vi "Test JSON config.vi"(0 "request cluster":variant, 1 "command description":string, 2 "command":string, 5 "<JSON> request documentation":string, 7 "response cluster":variant, 9 "<JSON> response documentation":string, 11 "error in (no error)":errorcluster) -> (4 "<JSON> API documentation":string, 15 "error out":errorcluster)   [LabVIEW 2019, in "Instrument.lvlib" / "Instrument.lvclass"]
uses:
  Instrument.lvclass
  ca868cea-1423-40d0-bede-52914c02769a.vi
  47e4b0b2-8925-4823-9c6b-443795284c27.vi
  <vilib>/JDP Science/JSONtext/Variant to JSON Text.vi
  <vilib>/JDP Science/JSONtext/LVClass Serializer/JSONtext LVClass Serializer.lvclass
  <vilib>/JDP Science/JSONtext/JSONtext.lvlib
  subsystems/Help/Help.lvclass
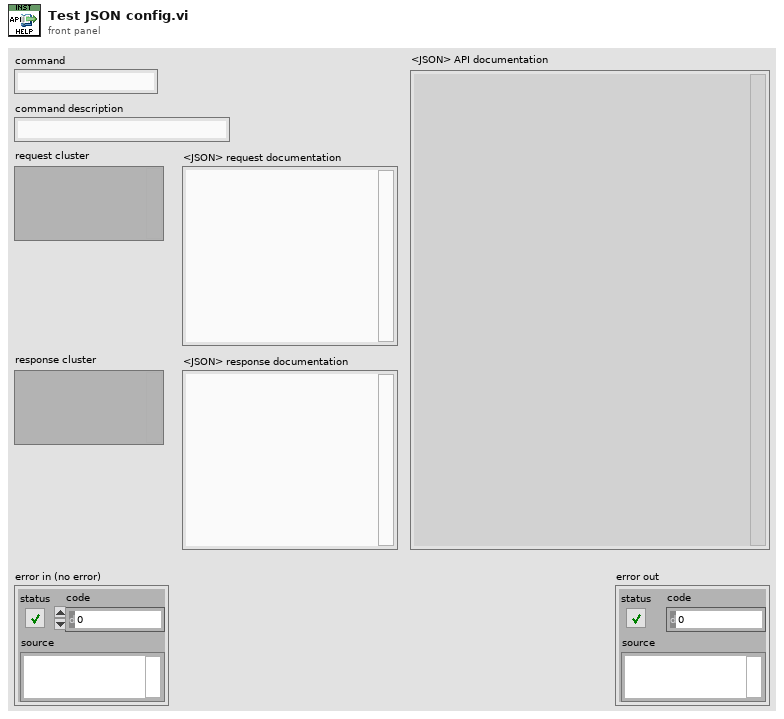
[diagram p1: front panel]
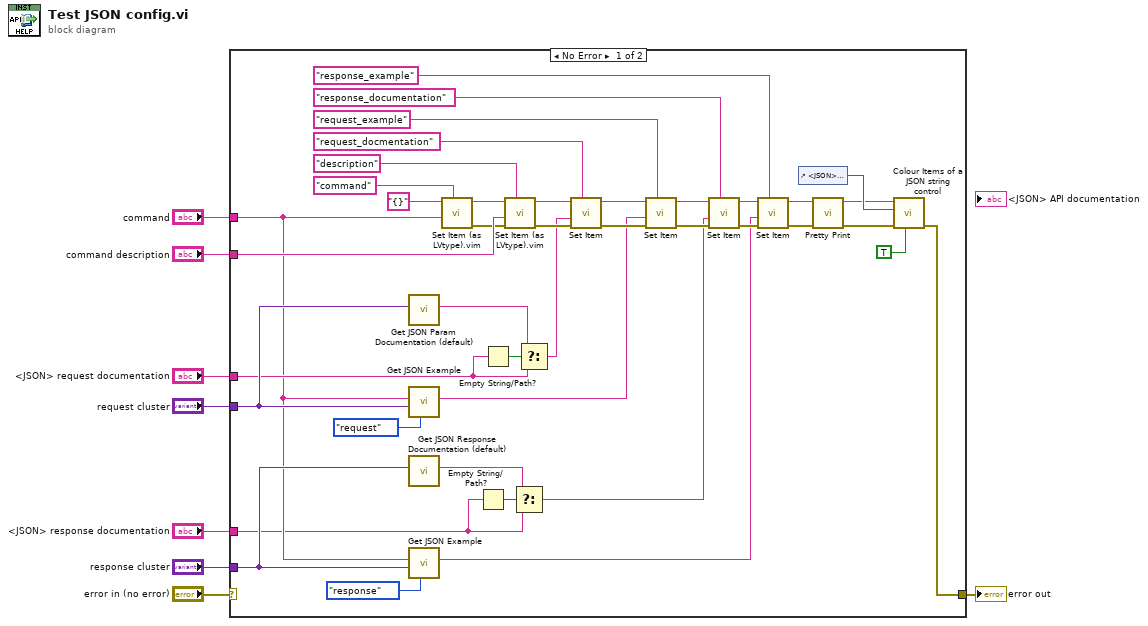
[diagram p0: block diagram]
diagram:
  n1 = case shown="No Error" "error in (no error)" {
    selector: "error in (no error)" -> [_ w49]
    tunnel: "command" -> [w14 _]
    tunnel: "command description" -> [w27 _]
    tunnel: "request cluster" -> [w41 _]
    tunnel: "<JSON> request documentation" -> [w38 _]
    tunnel: [w28 w49] -> w4
    tunnel: "response cluster" -> [w15 _]
    tunnel: "<JSON> response documentation" -> [w9 _]
    frame No Error {
      n2 = call "Get JSON Param Documentation (default).vi"("request cluster"=w41) -> ("<JSON> Request Documentation"=w40:string)  [unwired: 9 in, 1 out]
      n3 = call "Get JSON Example.vi"("type"=enum16{"request", "response"}."request", "params or result"=w41, "method"=w14) -> ("<JSON>"=w16:string)  [unwired: 7 in, 1 out]
      n4 = call "Get JSON Response Documentation (default).vi"("response cluster"=w15) -> ("<JSON> Response Documentation"=w12:string)  [unwired: 9 in, 1 out]
      n5 = call "Get JSON Example.vi"("type"=enum16{"request", "response"}."response", "params or result"=w15, "method"=w14) -> ("<JSON>"=w11:string)  [unwired: 7 in, 1 out]
      n6 = call "Set Item (as LVtype).vim"("$Path or Item Name"="command", "Anything"=w14, "JSON"="{}") -> ("error out"=w23:errorcluster, "<JSON>"=w26:string)  [unwired: 5 in, 1 out]
      n7 = Empty String/Path?(string/path=w9) -> (empty?=w13:bool)
      n8 = Empty String/Path?(string/path=w38) -> (empty?=w39:bool)
      n9 = call "Set Item (as LVtype).vim"("$Path or Item Name"="description", "error in (no error)"=w23, "Anything"=w27, "JSON"=w26) -> ("error out"=w42:errorcluster, "<JSON>"=w43:string)  [unwired: 4 in, 1 out]
      n10 = Select(t=w12, s=w13, f=w9) -> (s? t:f=w10:string)
      n11 = Select(t=w40, s=w39, f=w38) -> (s? t:f=w19:string)
      n12 = call <vilib>:"Set Item.vi"("$Path or Item Name"="request_docmentation", "error in (no error)"=w42, "JSON to Insert"=w19, "JSON"=w43) -> ("error out"=w33:errorcluster, "<JSON>"=w34:string)  [unwired: 4 in, 1 out]
      n13 = call <vilib>:"Set Item.vi"("$Path or Item Name"="request_example", "error in (no error)"=w33, "JSON to Insert"=w16, "JSON"=w34) -> ("error out"=w31:errorcluster, "<JSON>"=w32:string)  [unwired: 4 in, 1 out]
      n14 = call <vilib>:"Set Item.vi"("$Path or Item Name"="response_documentation", "error in (no error)"=w31, "JSON to Insert"=w10, "JSON"=w32) -> ("error out"=w36:errorcluster, "<JSON>"=w35:string)  [unwired: 4 in, 1 out]
      n15 = call <vilib>:"Set Item.vi"("$Path or Item Name"="response_example", "error in (no error)"=w36, "JSON to Insert"=w11, "JSON"=w35) -> ("error out"=w21:errorcluster, "<JSON>"=w22:string)  [unwired: 4 in, 1 out]
      n16 = control-ref of="<JSON> API documentation"() -> (w48:refnum<vi>)
      n17 = call <vilib>:"Pretty Print.vi"("error in (no error)"=w21, "JSON"=w22) -> ("error out"=w46:errorcluster, "<JSON>"=w20:string)  [unwired: 7 in, 1 out]
      n18 = call <vilib>:"Colour Items of a JSON string control.vi"("Defer Panel Updates"=TRUE, "error in (no error)"=w46, "String Control"=w48, "JSON"=w20) -> ("error out"=w28:errorcluster)  [unwired: 7 in]
    }
    frame Error {
    }
  }
  "error out" <- w4
